vi "A Distance to Angle.vi"() -> (3 "Angle":dbl)   [LabVIEW 2015]
uses:
  Robot Global Data.vi
panel:
  out "Vision Data":T1
  out "Distance":dbl
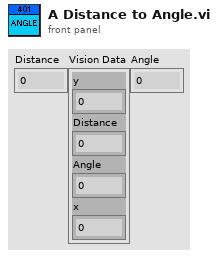
[diagram p1: front panel]
types:
  T1 = cluster{"y":dbl, "Distance":dbl, "Angle":dbl, "x":dbl}
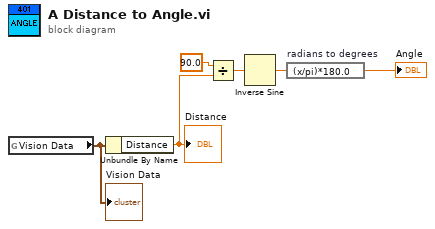
[diagram p0: block diagram]
diagram:
  n1 = global read "Robot Global Data.vi" "Vision Data"() -> (w2:T1)
  "Vision Data" <- w2
  n2 = Unbundle By Name(w2) -> ("Distance"=w1:dbl)
  "Distance" <- w1
  n3 = Divide(x=90.0 ("y"), y=w1) -> (x/y=w6:dbl)
  n4 = Inverse Sine(1:w6) -> (0:w5:dbl)
  n5 = expression code="(x/pi)*180.0" "radians to degrees"(w5) -> (→"Angle":dbl)
